vi "SAV.vi"(8 "error in (no error)":errorcluster, 10 "Memory":T2, 11 "refnum in":T1) -> (0 "error out":errorcluster, 3 "refnum out":T1, 4 "question out":string)   [LabVIEW 2021, in "Korad KA3305P.lvlib"]
uses:
  Korad KA3305P.lvlib
  MemoryNo.ctl
  Reference.ctl
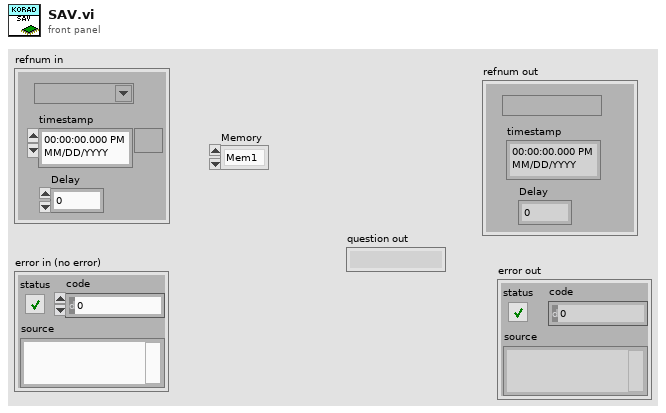
[diagram p1: front panel]
types:
  T1 = typedef "Korad KA3305P.lvlib/Reference.ctl" = cluster{"refnum":refnum<visa-resource-name>, "timestamp":timestamp, "Delay":dbl}
  T2 = typedef "Korad KA3305P.lvlib/MemoryNo.ctl" = enum16{"Mem1", "Mem2", "Mem3", "Mem4", "Mem5"}
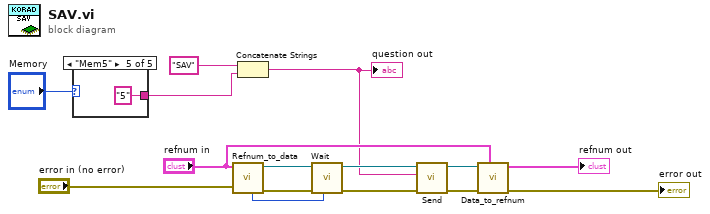
[diagram p0: block diagram]
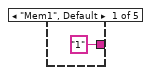
[diagram p2: hidden frame]
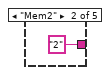
[diagram p3: hidden frame]
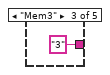
[diagram p4: hidden frame]
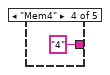
[diagram p5: hidden frame]
diagram:
  n1 = case shown="\"Mem5\"" "Memory" {
    tunnel: ["1" ("string") "2" ("string") "3" ("string") "4" ("string") "5" ("string")] -> w15
    frame "Mem1", Default {
    }
    frame "Mem2" {
    }
    frame "Mem3" {
    }
    frame "Mem4" {
    }
    frame "Mem5" {
    }
  }
  n2 = call "Refnum_to_data.vi"("error in (no error)"="error in (no error)", "refnum in"="refnum in") -> ("error out"=w7:errorcluster, "DAQ refnum out"=w8:refnum<visa-resource-name>, "delay out"=w9:u32)  [unwired: 7 in]
  n3 = Concatenate Strings("SAV" ("string"), w15) -> (w2:string)
  "question out" <- w2
  n4 = call "Wait.vi"("milliseconds to wait"=w9, "error in (no error)"=w7, "refnum in"=w8) -> ("error out"=w3:errorcluster, "refnum out"=w5:refnum<visa-resource-name>)  [unwired: 7 in]
  n5 = call "Send.vi"("error in (no error)"=w3, "data"=w2, "refnum in"=w5) -> ("error out"=w6:errorcluster, "refnum out"=w11:refnum<visa-resource-name>)  [unwired: 7 in]
  n6 = call "Data_to_refnum.vi"("refnum in"="refnum in", "error in (no error)"=w6, "DAQ refnum in"=w11) -> ("error out"=→"error out":errorcluster, "refnum out"=→"refnum out":T1)  [unwired: 7 in]
